vi "Configure Signal Input.vi"(7 "Wide Reserve (T: Automatically)":bool=TRUE, 8 "Error In (no error)":errorcluster, 9 "Signal Input Impedance (0:50 ohm)":u16(ring) items=["50 ohm", "1 Mohm"], 10 "Mode (0: High Reserve)":u16(ring) items=["High Reserve", "Normal ", "Low Noise"], 11 "VISA Resource Name":refnum<visa-resource-name>) -> (0 "Error Out":errorcluster, 3 "VISA Resource Name Out":refnum<visa-resource-name>)   [LabVIEW 2010, in "Stanford Research 844.lvlib"]
doc: "This VI configures signal input."
uses:
  <instrlib>/Stanford Research 844/Stanford Research 844.lvlib
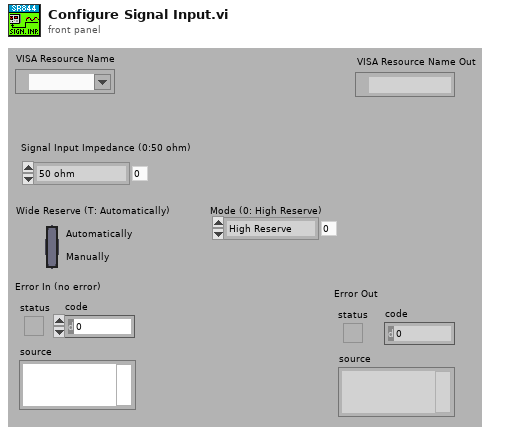
[diagram p1: front panel]
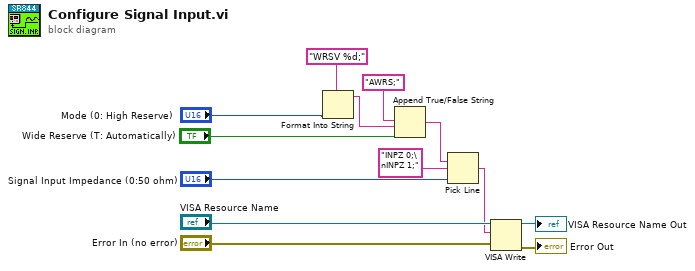
[diagram p0: block diagram]
diagram:
  n1 = Format Into String(format string="WRSV %d;" ("multi-line string"), "Mode (0: High Reserve)") -> (resulting string=w5:string)  [unwired: 2 in, 1 out]
  n2 = Append True/False String(1:"Wide Reserve (T: Automatically)", 2:w5, 3:"AWRS;" ("write buffer (\"\")")) -> (0:w1:string)  [unwired: 1 in]
  n3 = Pick Line(string ("")=w1, multi-line string="INPZ 0;\nINPZ 1;", line index="Signal Input Impedance (0:50 ohm)") -> (output string=w4:string)
  n4 = VISA Write(VISA resource name="VISA Resource Name", write buffer=w4, error in (no error)="Error In (no error)") -> (VISA resource name out=→"VISA Resource Name Out":refnum<visa-resource-name>, error out=→"Error Out":errorcluster)  [unwired: 1 out]
